vi "Check NewStateNotify is Registered.vi"(8 "error in (no error)":errorcluster, 11 "CSM-Helper in":refnum<class "CSM-Helper.lvclass">) -> (0 "error out":errorcluster, 2 "NewStateNotify Registed":bool, 3 "CSM-Helper out":refnum<class "CSM-Helper.lvclass">)   [LabVIEW 2020, in "CSM-Helper.lvclass"]
uses:
  CSM-Helper.lvclass
  CSM-Helper.lvclass/CSM-Helper.ctl
  Properties/Read Event Structure Ref.vi
  23d72305-f0a8-4ea4-80e2-b48919ab28b1.vi
  ef047b75-69a1-48c7-876b-f6f5e73956db.vi
  <userlib>/_NEVSTOP/Communicable State Machine(CSM)/Communicable State Machine.lvlib
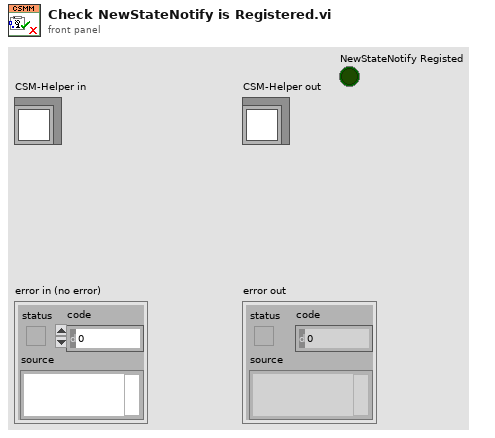
[diagram p1: front panel]
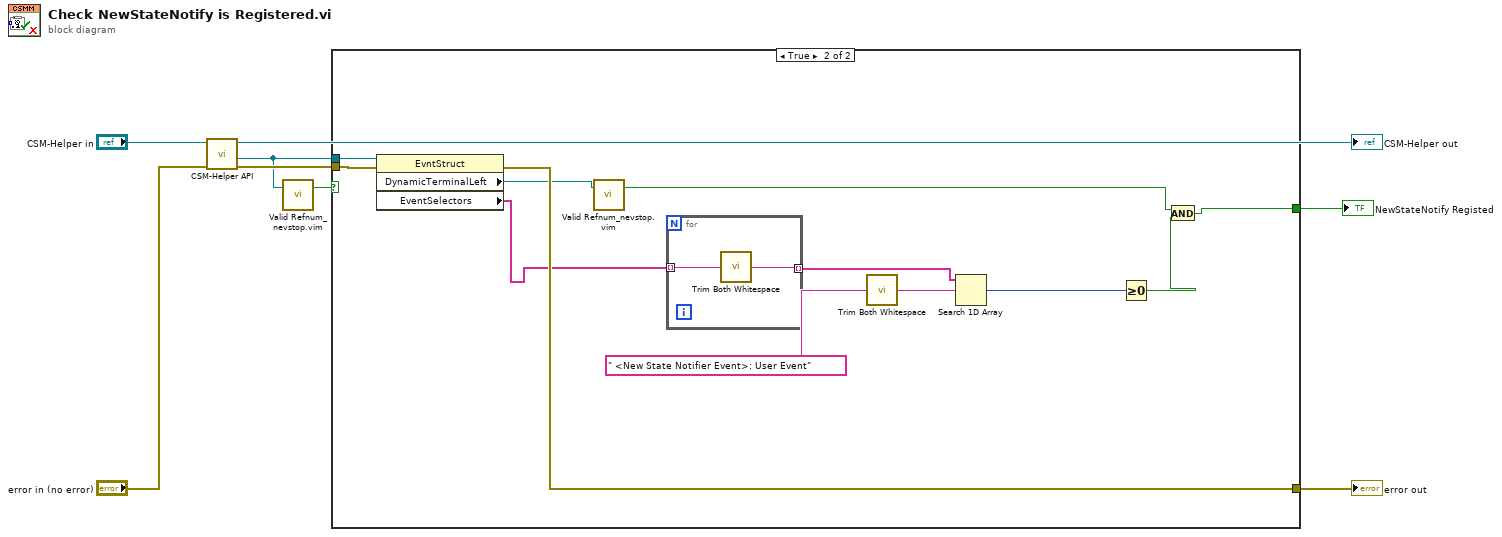
[diagram p0: block diagram]
diagram:
  n1 = call-poly "CSM-Helper API.vi"("error in (no error)"="error in (no error)", "CSM-Helper in"="CSM-Helper in") -> ("error out"=w5:errorcluster, "Event Structure"=w3:refnum<vi>, "CSM-Helper out"=→"CSM-Helper out":refnum<class "CSM-Helper.lvclass">)  [unwired: 7 in]
  n2 = call "Valid Refnum_nevstop.vim"("number/path/refnum"=w3) -> ("Valid Number/Path/Refnum"=w2:bool)  [unwired: 2 in]
  n3 = case shown="True" w2 {
    tunnel: w5 -> [w9 w21]
    tunnel: [w9 w20] -> w4
    tunnel: w3 -> [_ w19]
    tunnel: [_ w10] -> w1
    frame False {
    }
    frame True {
      n4 = property class="EvntStruct"(reference=w19, error in=w21) -> (error out=w20:errorcluster, "DynamicTerminalLeft"=w18:refnum<vi>, "EventSelectors"=w13:string[])  [unwired: 1 out]
      n5 = call "Valid Refnum_nevstop.vim"("number/path/refnum"=w18) -> ("Valid Number/Path/Refnum"=w12:bool)  [unwired: 2 in]
      n6 = for {
        tunnel: [w22] -> w14 mode=indexing
        tunnel: w13 -> [w23] mode=indexing
        n7 = call <userlib>:"Trim Both Whitespace.vi"("string"=w23) -> ("trimmed string"=w22:string)  [unwired: 1 in]
      }
      n8 = call <userlib>:"Trim Both Whitespace.vi"("string"=" <New State Notifier Event>: User Event" ("element")) -> ("trimmed string"=w15:string)  [unwired: 1 in]
      n9 = Search 1D Array(1D array=w14, element=w15) -> (index of element=w17:i32)  [unwired: 1 in]
      n10 = Greater Or Equal To 0?(x=w17) -> (x >= 0?=w11:bool)
      n11 = And(x=w12, y=w11) -> (x .and. y?=w10:bool)
    }
  }
  "error out" <- w4
  "NewStateNotify Registed" <- w1
